vi "TCPIP_SERVEUR.vi"() -> ()   [LabVIEW 2018]
panel:
  out "Numeric":dbl
  out "String 2":string
  out "String":string
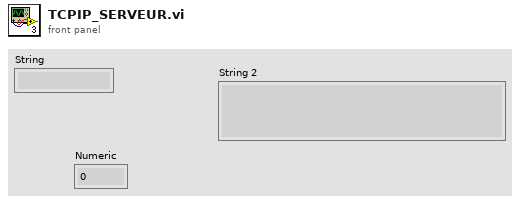
[diagram p1: front panel]
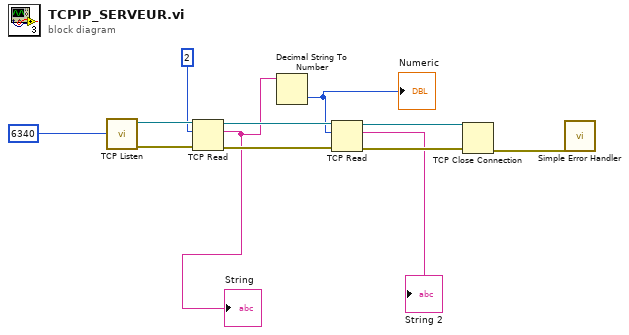
[diagram p0: block diagram]
diagram:
  n1 = call <vilib>:"TCP Listen.vi"("port"=6340) -> ("error out"=w9:errorcluster, "connection ID"=w11:refnum<k5>)  [unwired: 6 in, 3 out]
  n2 = TCP Read(connection ID=w11, bytes to read=2, error in (no error)=w9) -> (connection ID out=w8:refnum<k5>, data out=w2:string, error out=w7:errorcluster)  [unwired: 2 in]
  "String" <- w2
  n3 = Decimal String To Number(string=w2) -> (number=w1:i32)  [unwired: 2 in, 1 out]
  "Numeric" <- w1
  n4 = TCP Read(connection ID=w8, bytes to read=w1, error in (no error)=w7) -> (connection ID out=w5:refnum<k5>, data out=→"String 2":string, error out=w6:errorcluster)  [unwired: 2 in]
  n5 = TCP Close Connection(connection ID=w5, error in (no error)=w6) -> (error out=w10:errorcluster)  [unwired: 1 in, 1 out]
  n6 = call <vilib>:"Simple Error Handler.vi"("error in (no error)"=w10) -> ()  [unwired: 4 in, 5 out]
